vi "Apply Perspective to Image.vi"(7 "File Path (Image Calibration)":path=path "C:/Users/whitemrj/Desktop/New folder/pizza cal.png", 8 "error in":errorcluster, 10 "Image in":T1, 11 "Image Name":string="untitled") -> (0 "error out":errorcluster, 2 "Image out":T1)   [LabVIEW 2012]
uses:
  <vilib>/vision/Image Controls.llb/IMAQ Image.ctl
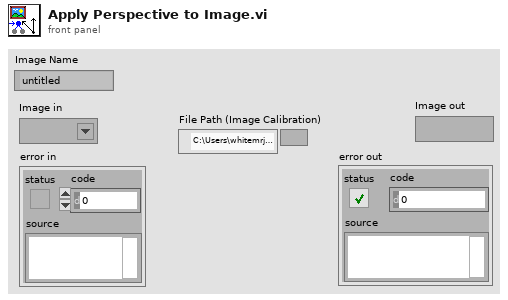
[diagram p1: front panel]
types:
  T1 = typedef "IMAQ Image.ctl" = refnum<image>
  T2 = typedef "Image Type" = u32
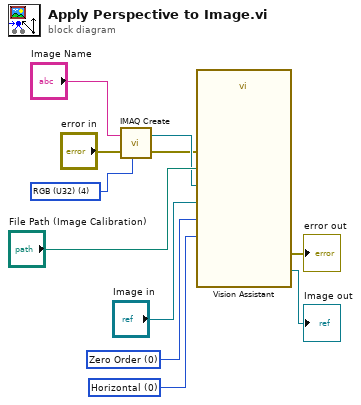
[diagram p0: block diagram]
diagram:
  w1 = T2 4 items=["Grayscale (U8)", "Grayscale (I16)", "Grayscale (SGL)", "Complex (CSG)", "RGB (U32)", "HSL (U32)", "RGB (U64)", "Grayscale (U16)"] ("Image Type")
  w6 = u32 0 items=["Horizontal", "Vertical", "Central", "1st Diagonal", "2nd Diagonal"] ("Type of Symmetry (Geometry 1)")
  w9 = u32 0 items=["Zero Order", "Bi-Linear", "Quadratic", "Cubic Spline"] ("Interpolation Type (Image Correction 1)")
  n1 = call "IMAQ Create"("Image Name"="Image Name", "Image Type"=w1, "error in (no error)"="error in") -> ("New Image"=w5:T1, "error out"=w2:errorcluster)  [unwired: 2 in]
  n2 = call "Vision Assistant"("Image In"="Image in", "File Path (Image Calibration 1)"="File Path (Image Calibration)", "Interpolation Type (Image Correction 1)"=w9, "Image Dst"=w5, "Type of Symmetry (Geometry 1)"=w6, "error in"=w2) -> ("Image Out"=→"Image out":T1, "error out"=→"error out":errorcluster)  [unwired: 20 in]
